vi "Get Node Details.vi"(8 "error in (no error)":errorcluster, 11 "Node Refnum":refnum<vi>) -> (0 "error out":errorcluster, 3 "output cluster":T1)   [LabVIEW 2014, in "SmartPalette.lvlib"]
uses:
  SmartPalette.lvlib
  Controls/GObjectDetail.ctl
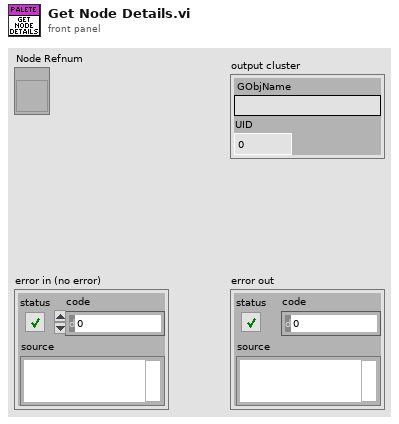
[diagram p1: front panel]
types:
  T1 = typedef "SmartPalette.lvlib/GObjectDetail.ctl" = cluster{"GObjName":string, "UID":i32}
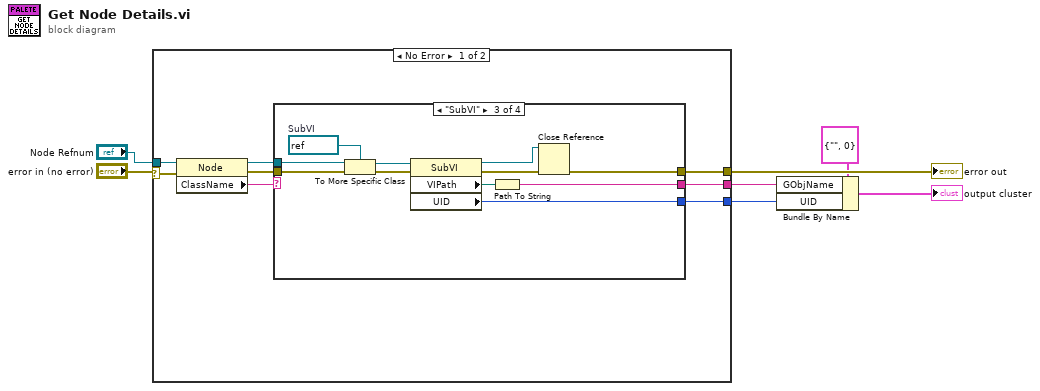
[diagram p0: block diagram]
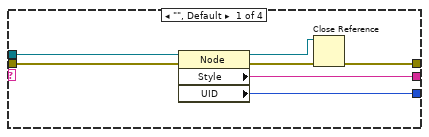
[diagram p2: hidden frame]
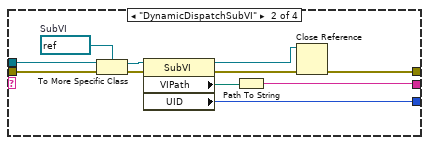
[diagram p3: hidden frame]
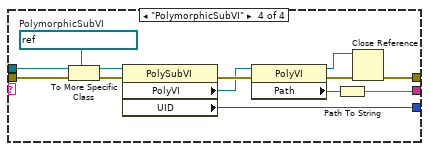
[diagram p4: hidden frame]
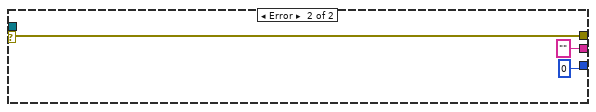
[diagram p5: hidden frame]
diagram:
  n1 = case shown="No Error" "error in (no error)" {
    selector: "error in (no error)" -> [w14 w60]
    tunnel: "Node Refnum" -> [w15 _]
    tunnel: [w12 w60] -> w5
    tunnel: [w9 "" ("Style")] -> w2
    tunnel: [w8 0 ("UID")] -> w1
    frame No Error {
      n2 = property class="Node"(reference=w15, error in=w14) -> (reference out=w10:refnum<vi>, error out=w13:errorcluster, "ClassName"=w11:string)
      n3 = case shown="\"SubVI\"" w11 {
        tunnel: w13 -> [w22 w30 w41 w57]
        tunnel: [w18 w25 w37 w49] -> w12
        tunnel: w10 -> [w21 w29 w34 w45]
        tunnel: [w20 w27 w39 w47] -> w9
        tunnel: [w16 w23 w35 w46] -> w8
        frame "", Default {
          n4 = property class="Node"(reference=w21, error in=w22) -> (reference out=w17:refnum<vi>, error out=w19:errorcluster, "Style"=w20:string, "UID"=w16:i32)
          n5 = Close Reference(reference=w17, error in (no error)=w19) -> (error out=w18:errorcluster)
        }
        frame "DynamicDispatchSubVI" {
          w31 = refnum<vi> refnum  # SubVI
          n6 = To More Specific Class(target class=w31, reference=w29, error in=w30) -> (specific class reference=w32:refnum<vi>, error out=w33:errorcluster)
          n7 = property class="SubVI"(reference=w32, error in=w33) -> (reference out=w24:refnum<vi>, error out=w26:errorcluster, "VIPath"=w28:path, "UID"=w23:i32)
          n8 = Path To String(path=w28) -> (string=w27:string)
          n9 = Close Reference(reference=w24, error in (no error)=w26) -> (error out=w25:errorcluster)
        }
        frame "SubVI" {
          w43 = refnum<vi> refnum  # SubVI
          n10 = To More Specific Class(target class=w43, reference=w34, error in=w41) -> (specific class reference=w44:refnum<vi>, error out=w40:errorcluster)
          n11 = property class="SubVI"(reference=w44, error in=w40) -> (reference out=w36:refnum<vi>, error out=w38:errorcluster, "VIPath"=w42:path, "UID"=w35:i32)
          n12 = Path To String(path=w42) -> (string=w39:string)
          n13 = Close Reference(reference=w36, error in (no error)=w38) -> (error out=w37:errorcluster)
        }
        frame "PolymorphicSubVI" {
          w55 = refnum<vi> refnum  # PolymorphicSubVI
          n14 = To More Specific Class(target class=w55, reference=w45, error in=w57) -> (specific class reference=w54:refnum<vi>, error out=w56:errorcluster)
          n15 = property class="PolySubVI"(reference=w54, error in=w56) -> (error out=w53:errorcluster, "PolyVI"=w51:refnum<vi>, "UID"=w46:i32)  [unwired: 1 out]
          n16 = property class="PolyVI"(reference=w51, error in=w53) -> (reference out=w48:refnum<vi>, error out=w52:errorcluster, "Path"=w50:path)
          n17 = Path To String(path=w50) -> (string=w47:string)
          n18 = Close Reference(reference=w48, error in (no error)=w52) -> (error out=w49:errorcluster)
        }
      }
    }
    frame Error {
    }
  }
  "error out" <- w5
  n19 = Bundle By Name(cluster=T1 {"GObjName"="", "UID"=0} ("GobjDetails"), "GObjName"=w2, "UID"=w1) -> (→"output cluster":T1)
